vi "Do.vi"(8 "error in (no error)":errorcluster, 10 "Actor in":refnum<class "Actor.lvclass">, 11 "InitializeReport Msg":refnum<class "InitializeReport Msg.lvclass">) -> (0 "error out":errorcluster, 2 "Actor out":refnum<class "Actor.lvclass">)   [LabVIEW 2019, in "LocalReport.lvlib" / "InitializeReport Msg.lvclass"]
doc: "This VI delivers the message to the actor by calling the appropriate method(s) on the actor."
uses:
  InitializeReport Msg.lvclass
  <vilib>/ActorFramework/Actor/Actor.lvclass
  LocalReport/LocalReport.lvclass
  C:/Program Files (x86)/National Instruments/LabVIEW 2019/vi.lib/ActorFramework/Actor/Actor.lvclass
  InitializeReport Msg.lvclass/InitializeReport Msg.ctl
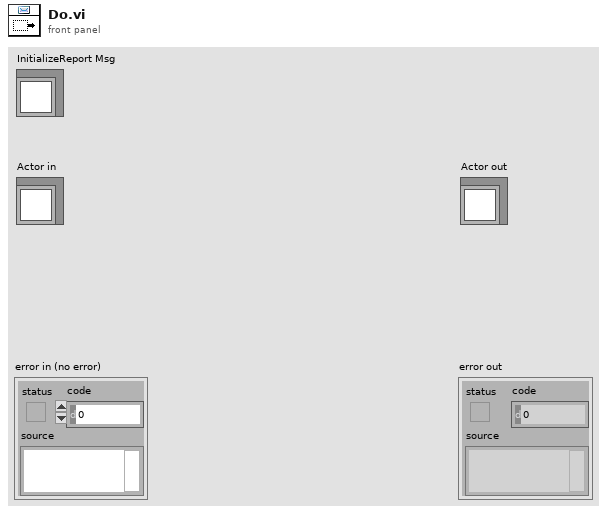
[diagram p1: front panel]
types:
  T1 = cluster{"Report Path":path, "Report  Format":enum16{"CSV", "XML", "PDF", "Excel", "TXT"}, "Enabled State":bool, "Customer name":string}
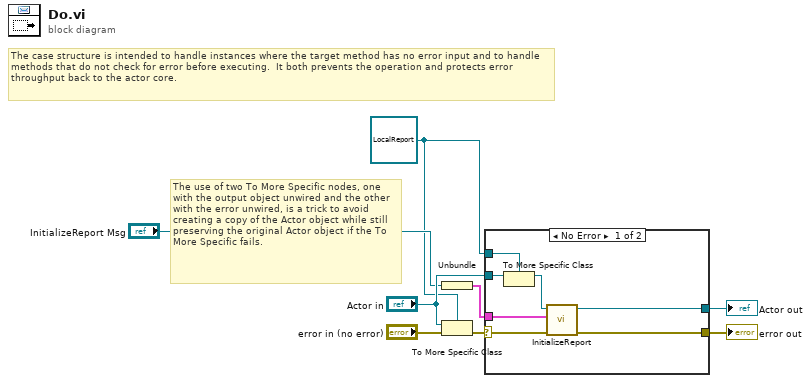
[diagram p0: block diagram]
diagram:
  w3 = refnum<class "LocalReport.lvclass"> refnum ("Actor in")
  # "The use of two To More Specific nodes, one with the output object unwired and the other with the error unwired, is a trick to avoid creating a copy of the Actor object while still preserving the original Actor object if the To More Specific fails."
  # "The case structure is intended to handle instances where the target method has no error input and to handle methods that do not check for error before executing.  It both prevents the operation and protects error throughput back to the actor core."
  n1 = Unbundle("InitializeReport Msg") -> (w1:T1)
  n2 = To More Specific Class(target class=w3, reference="Actor in", error in="error in (no error)") -> (error out=w2:errorcluster)  [unwired: 1 out]
  n3 = case shown="No Error" w2 {
    selector: w2 -> [w13 w17]
    tunnel: [w15 w17] -> w8
    tunnel: [w14 w16] -> w7
    tunnel: "Actor in" -> [w12 w16]
    tunnel: w3 -> [w11 _]
    tunnel: w1 -> [w9 _]
    frame No Error {
      n4 = To More Specific Class(target class=w11, reference=w12) -> (specific class reference=w10:refnum<class "LocalReport.lvclass">)  [unwired: 1 in, 1 out]
      n5 = call-dynamic "InitializeReport.vi"("error in (no error)"=w13, "Local Report Parameter"=w9, "LocalReport in"=w10) -> ("error out"=w15:errorcluster, "LocalReport out"=w14:refnum<class "LocalReport.lvclass">)  [unwired: 7 in]
    }
    frame Error {
      # "If type check fails, pass the original object out again."
    }
  }
  "error out" <- w8
  "Actor out" <- w7
